vi "Find Command with Tag.vi"(10 "Command Tag":string, 11 "Commands":cluster{"Time (s)":dbl, T1, bool}[](array[cluster])) -> (1 "Index":i32, 2 "Found Command":cluster{"Time (s)":dbl, T1, bool}={"Time (s)"=0.0, {"Name"="", "CPTM.DataType"=variant, "All Control Values Variant"=[], "icon full"={"image type"=0, "image depth"=0, "image"=[], "mask"=[], "colors"=[], "Rectangle"={"left"=0, "top"=0, "right"=0, "bottom"=0}}, "icon scaled"={"image type"=0, "image depth"=0, "image"=[], "mask"=[], "colors"=[], "Rectangle"={"left"=0, "top"=0, "right"=0, "bottom"=0}}, "Path"=path "", "Subsystem Color"=16777216}, FALSE}, 3 "Found":bool)   [LabVIEW 2025]
uses:
  Types/Single Cmd Info.ctl
  <vilib>/picture/picture.llb/imagedata.ctl
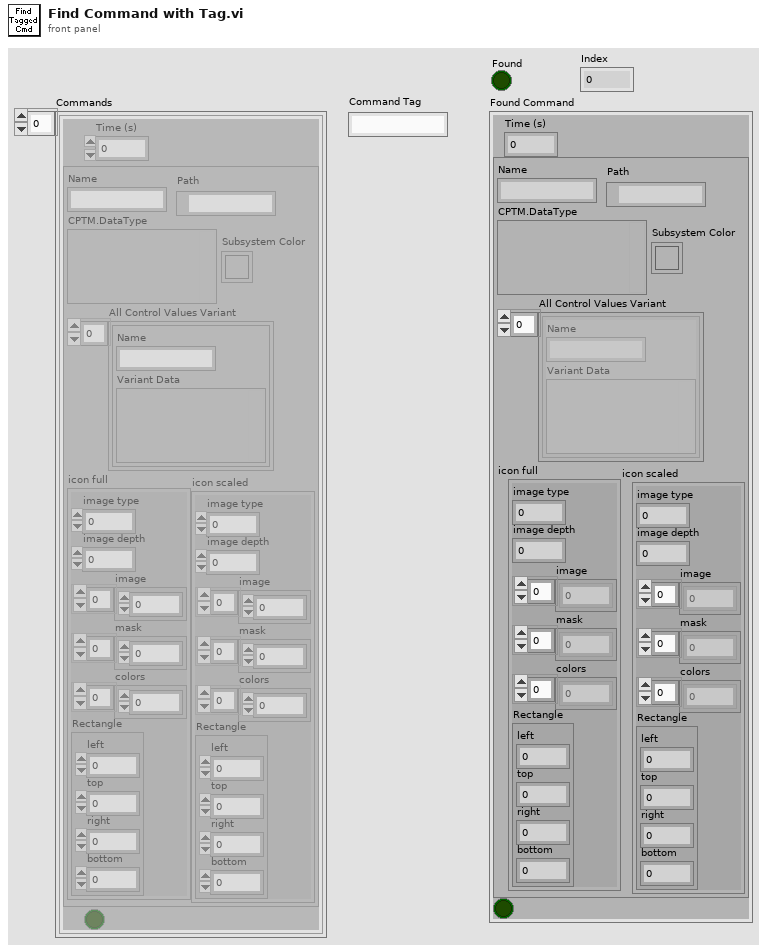
[diagram p1: front panel]
types:
  T1 = typedef "Single Cmd Info.ctl" = cluster{"Name":string, "CPTM.DataType":variant, "All Control Values Variant":cluster{"Name":string, "Variant Data":variant}[], "icon full":T2, "icon scaled":T2, "Path":path, "Subsystem Color":u32}
  T2 = typedef "imagedata.ctl" = cluster{"image type":i32, "image depth":i32, "image":u8[], "mask":u8[], "colors":u32[], "Rectangle":cluster{"left":i16, "top":i16, "right":i16, "bottom":i16}}
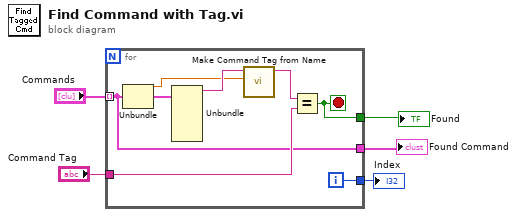
[diagram p0: block diagram]
diagram:
  n1 = for {
    tunnel: "Commands" -> [w7] mode=indexing
    tunnel: "Command Tag" -> [w9]
    tunnel: [w8] -> w3
    tunnel: [w7] -> w2
    tunnel: [w6] -> w1
    i -> [w6]
    stop <- w8 stop-if-true
    n2 = Unbundle(w7) -> ("Time (s)"=w10:dbl, w13:T1)  [unwired: 1 out]
    n3 = Unbundle(w13) -> ("Name"=w11:string)  [unwired: 6 out]
    n4 = call "Make Command Tag from Name.vi"("Time"=w10, "Cmd Name"=w11) -> ("Cmd Tag"=w12:string)  [unwired: 9 in]
    n5 = Equal?(x=w12, y=w9) -> (x = y?=w8:bool)
  }
  "Found" <- w3
  "Found Command" <- w2
  "Index" <- w1
